vi "buffer changed data.vi"(0 "Serial port asssistant model in":refnum<class "Serial port assistant model.lvclass">, 7 "changed data":string, 11 "error in (no error)":errorcluster) -> (4 "Serial port asssistant model out":refnum<class "Serial port assistant model.lvclass">, 15 "error out":errorcluster)   [LabVIEW 2022 SP3, in "Serial port assistant model.lvlib" / "Serial port assistant model.lvclass"]
uses:
  Serial port assistant model.lvclass
  changed data--type.ctl
  Serial port assistant model.lvclass/Serial port assistant model.ctl
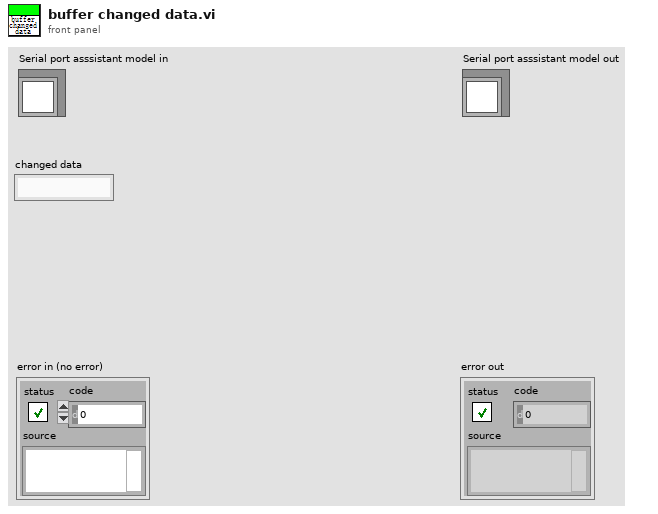
[diagram p1: front panel]
types:
  T1 = typedef "Serial port assistant model.lvlib/Serial port assistant model.lvclass/changed data--type.ctl" = cluster{"changed data":string}
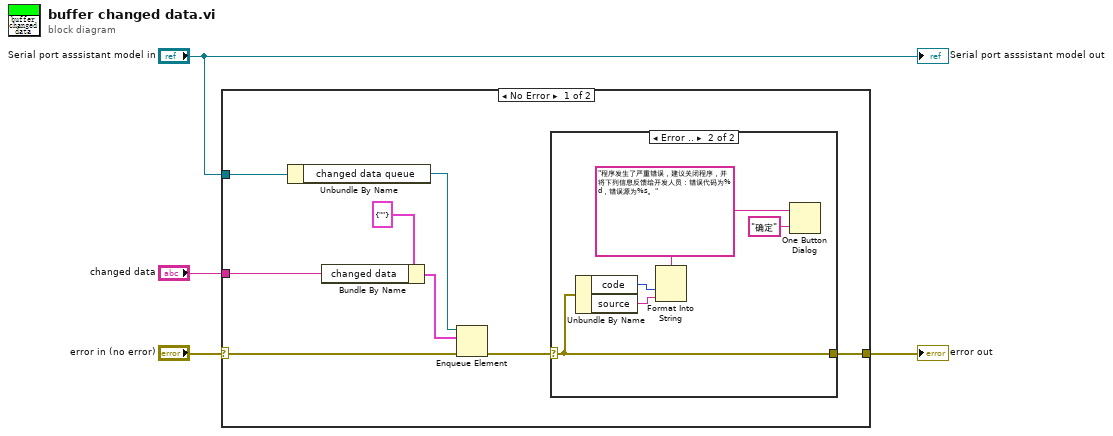
[diagram p0: block diagram]
diagram:
  n1 = case shown="No Error" "error in (no error)" {
    selector: "error in (no error)" -> [w7 w19]
    tunnel: "Serial port asssistant model in" -> [w12 _]
    tunnel: "changed data" -> [w11 _]
    tunnel: [w5 w19] -> w2
    frame No Error {
      n2 = Unbundle By Name(w12) -> ("changed data queue"=w10:refnum<queue>)
      n3 = Bundle By Name(cluster=T1 {"changed data"=""} ("element"), "changed data"=w11) -> (w8:T1)
      n4 = Enqueue Element(queue=w10, element=w8, error in (no error)=w7) -> (error out=w6:errorcluster)  [unwired: 1 in, 2 out]
      n5 = case shown="Error .." w6 {
        selector: w6 -> [w13 w14]
        tunnel: [w13 w14] -> w5
        frame No Error {
        }
        frame Error {
          w16 = "程序发生了严重错误，建议关闭程序，并将下列信息反馈给开发人员：错误代码为%d，错误源为%s。" ("format string")
          n6 = Unbundle By Name(w14) -> ("code"=w18:i32, "source"=w17:string)
          n7 = Format Into String(format string=w16, w18, w17) -> ()  [unwired: 2 in, 2 out]
          n8 = One Button Dialog(message=w16, button name ("OK")="确定") -> ()  [unwired: 1 out]
        }
      }
    }
    frame Error {
    }
  }
  "error out" <- w2
  "Serial port asssistant model out" <- "Serial port asssistant model in"
